vi "Own_Code_Light2_EV3.vi"() -> ()   [LabVIEW 2012]
uses:
  SubVIs/LVPresent_Globals.vi
panel:
  in  "Tab Control":enum32{"Page 1", "Page 2"}(tab)
  in  "Need a hint":bool
  in  "Open 2":bool
  in  "Ans. 4":bool
  in  "Ans. 3":bool
  in  "Back":bool
  # "Let's take a look at the color sensor...\n\nAttach the color sensor to the EV3 device, and write some code to have the robot stop on a black line. Press the Open button to start a new VI."
  # "Step 2: \n\nSave As your VI  and rename it. Then, start a new VI. Now, test out the colors feature on the light sensor. Write code that outputs the number that corresponds to the color value on the light sensor. Then, add in the Log Light (red) function. On default, this function records the color value every 0.5 seconds over 10 seconds.  Play around with this data logging function."
  # "Hint 1: Check out the functions under the Sensors tab  and the Timing  tab under Complete, I/O and MINDSTORMS Robotics. Remember that if you do not know what a function does, you can turn on Show Context Help, under the Help tab. \n\nHint 1b: Think about the difference between the light-colored floor and the black tape. \n\n\n\n\n\nMore information on the Log Light (red function): run this function parallel to the rest of the VI. This means that you do not need to connect the pink wire through this function. Also, to view this data afterwards, go to the Tools tab >> NXT/ EV3 Application Browser >> NXT/ EV3 Data Viewer and then click Launch. Then click Add Data and click on the NXT/ EV3 icon that looks identical to the Log Light (red) icon."
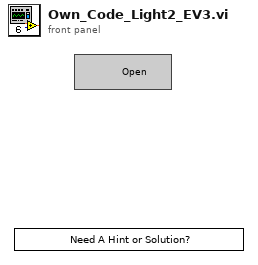
[diagram p1: front panel]
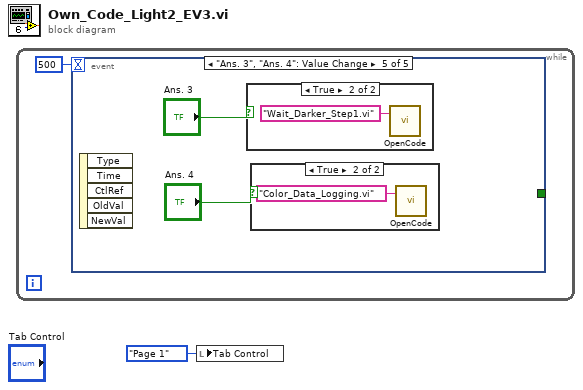
[diagram p0: block diagram]
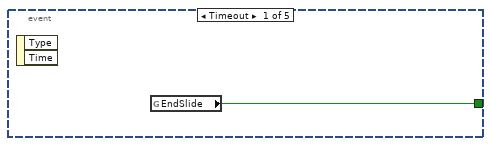
[diagram p2: hidden frame]
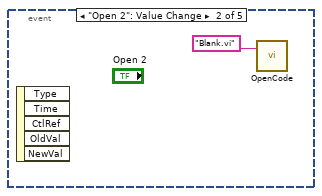
[diagram p3: hidden frame]
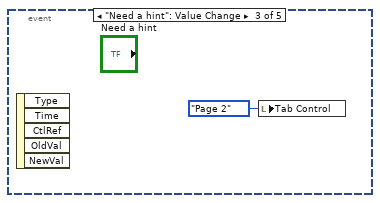
[diagram p4: hidden frame]
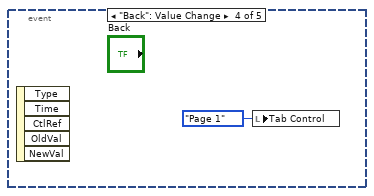
[diagram p5: hidden frame]
diagram:
  n1 = while {
    stop <- w3 stop-if-true
    n2 = event shown="[4] \"Ans. 3\", \"Ans. 4\": Value Change" {
      selector: _ -> [_ _ _ _ _]
      dyn-events: _ -> [_ _ _ _ _]
      timeout: 500 -> [_ _ _ _ _]
      tunnel: [w4 _ _ _ _] -> w3
      event Timeout {
        n3 = event-data() -> ()  [unwired: 1 in, 2 out]
        n4 = global read "LVPresent_Globals.vi" "EndSlide"() -> (w4:bool)
      }
      event "Open 2": Value Change {
        n5 = event-data() -> ()  [unwired: 1 in, 5 out]
        n6 = call "OpenCode.vi"("Code name"="Blank.vi") -> ()  [unwired: 3 in]
      }
      event "Need a hint": Value Change {
        n7 = event-data() -> ()  [unwired: 1 in, 5 out]
        n8 = local write "Tab Control"(enum32{"Page 1", "Page 2"}."Page 2" ("Tab Control")) -> ()
      }
      event "Back": Value Change {
        n9 = event-data() -> ()  [unwired: 1 in, 5 out]
        n10 = local write "Tab Control"(enum32{"Page 1", "Page 2"}."Page 1" ("Tab Control")) -> ()
      }
      event "Ans. 3", "Ans. 4": Value Change {
        n11 = event-data() -> ()  [unwired: 1 in, 5 out]
        n12 = case shown="True" "Ans. 3" {
          frame False {
          }
          frame True {
            n13 = call "OpenCode.vi"("Code name"="Wait_Darker_Step1.vi") -> ()  [unwired: 3 in]
          }
        }
        n14 = case shown="True" "Ans. 4" {
          frame False {
          }
          frame True {
            n15 = call "OpenCode.vi"("Code name"="Color_Data_Logging.vi") -> ()  [unwired: 3 in]
          }
        }
      }
    }
  }
  n16 = local write "Tab Control"(enum32{"Page 1", "Page 2"}."Page 1" ("Tab Control")) -> ()
